vi "Compare and Append Run.vi"(8 "error in (no error)":errorcluster, 9 "Repetitions":u32, 10 "Run":refnum<class "Run Instance.lvclass">, 11 "Schedule Cell in":refnum<class "Schedule Cell.lvclass">) -> (0 "error out":errorcluster, 1 "Cell Updated":bool, 2 "new Schedule Cell out":refnum<class "Schedule Cell.lvclass">, 3 "Schedule Cell out":refnum<class "Schedule Cell.lvclass">)   [LabVIEW 2020, in "CIRCUS_uServices.lvlib" / "Run Utilities.lvlib" / "Schedule Cell.lvclass"]
doc: "VI compares the Run Instance with the Cell. If they are the same, it updates the cell accordingly. Otherwise, it creates a new Cell"
uses:
  Schedule Cell.lvclass
  Run Instance/Run Instance.lvclass
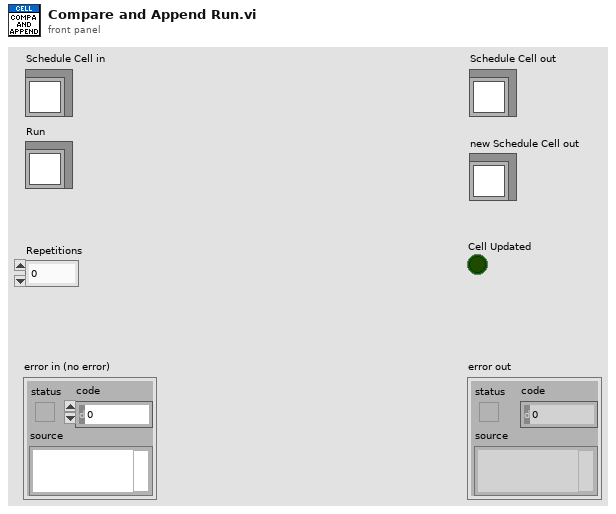
[diagram p1: front panel]
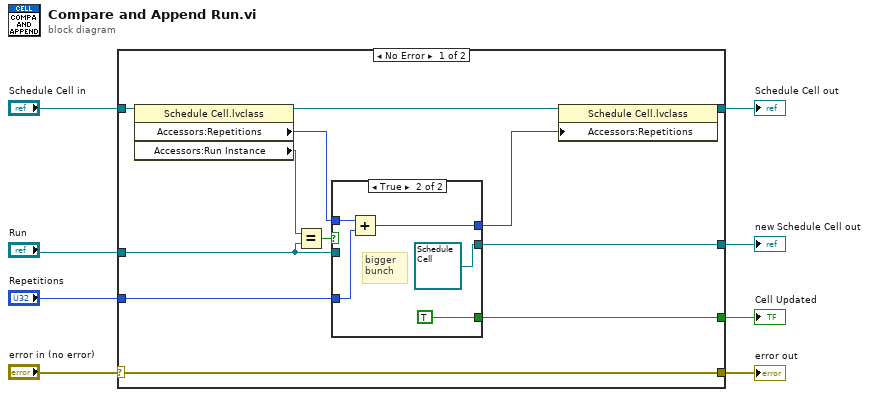
[diagram p0: block diagram]
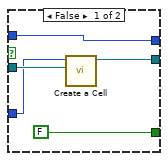
[diagram p2: hidden frame]
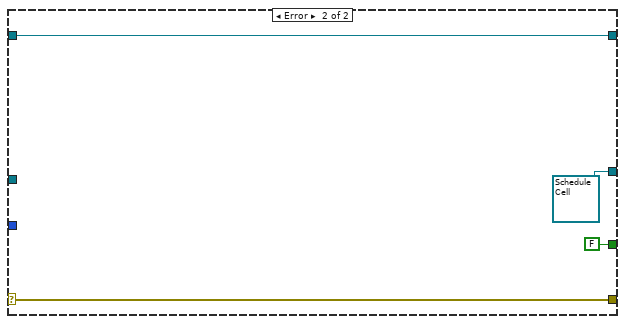
[diagram p3: hidden frame]
diagram:
  n1 = case shown="No Error" "error in (no error)" {
    selector: "error in (no error)" -> [w20 w34]
    tunnel: [w20 w34] -> w7
    tunnel: [w14 w33] -> w5
    tunnel: "Schedule Cell in" -> [w15 w33]
    tunnel: "Run" -> [w13 _]
    tunnel: "Repetitions" -> [w12 _]
    tunnel: [w11 refnum<class "Schedule Cell.lvclass"> refnum ("Schedule Cell out")] -> w2
    tunnel: [w10 FALSE] -> w1
    frame No Error {
      n2 = property class="Schedule Cell.lvclass"(reference=w15) -> (reference out=w9:refnum<class "Schedule Cell.lvclass">, "Accessors:Repetitions"=w18:u32, "Accessors:Run Instance"=w17:refnum<class "Run Instance.lvclass">)  [unwired: 1 in, 1 out]
      n3 = Equal?(x=w17, y=w13) -> (x = y?=w19:bool)
      n4 = case shown="True" w19 {
        tunnel: w13 -> [w24 _]
        tunnel: w18 -> [w25 w30]
        tunnel: [w25 w28] -> w16
        tunnel: [w22 refnum<class "Schedule Cell.lvclass"> refnum ("Schedule Cell out")] -> w11
        tunnel: w12 -> [w23 w29]
        tunnel: [FALSE ("Optimiser") TRUE] -> w10
        frame False {
          n5 = call "Create a Cell.vi"("Run Instance"=w24, "Repetitions"=w23) -> ("Schedule Cell out"=w22:refnum<class "Schedule Cell.lvclass">)  [unwired: 8 in, 1 out]
        }
        frame True {
          # "bigger bunch"
          n6 = Add(x=w30, y=w29) -> (x+y=w28:u32)
        }
      }
      n7 = property class="Schedule Cell.lvclass"(reference=w9, "Accessors:Repetitions"=w16) -> (reference out=w14:refnum<class "Schedule Cell.lvclass">)  [unwired: 1 in, 1 out]
    }
    frame Error {
    }
  }
  "error out" <- w7
  "Schedule Cell out" <- w5
  "new Schedule Cell out" <- w2
  "Cell Updated" <- w1
